vi "Set VI Ref.vi"(0 "reference in":refnum<class "Generic Utilities.lvclass">, 5 "error in (no error)":errorcluster, 6 "ReInit All to Default?":bool, 7 "GUI VI Ref":refnum<vi>, 8 "Initialize FP Control Refs":bool, 9 "Version #":string) -> (14 "reference out":refnum<class "Generic Utilities.lvclass">, 19 "error out":errorcluster)   [LabVIEW 2022 SP3, in "Generic Utilities.lvclass"]
uses:
  Generic Utilities.lvclass
  utils/FP Refnums.ctl
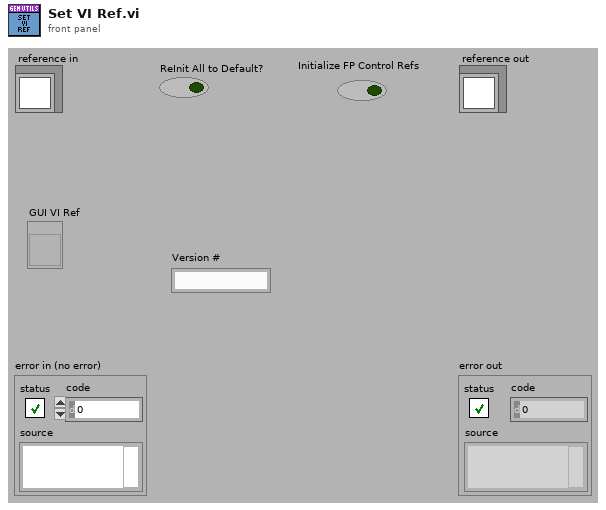
[diagram p1: front panel]
types:
  T1 = typedef "Generic Utilities.lvclass/FP Refnums.ctl" = cluster{"Panel refnum":refnum<vi>, "Control Labels":string[], "Refnums":refnum<vi>[]}
  T2 = typedef "Generic Utilities.lvclass/ObjectAttributesRef.ctl" = refnum<data-value>
  T3 = typedef "Generic Utilities.lvclass/ObjectAttributes.ctl" = cluster{"GUI Parameters":T4, "State Machine Control":cluster{"Timeout":i32, "State Queue":string[], "State History":string[], "State History Length":i32}, "Logging File Path":path, "OBJ not a refnum?":bool, "Timer Start":timestamp, "FP Refnums":T1}
  T4 = typedef "Generic Utilities.lvclass/GUI Parameters.ctl" = cluster{"Application Name":string, "GUI VI Ref":refnum<vi>, "Close Panel?":bool, "Message Window ref":refnum<vi>, "Version #":string}
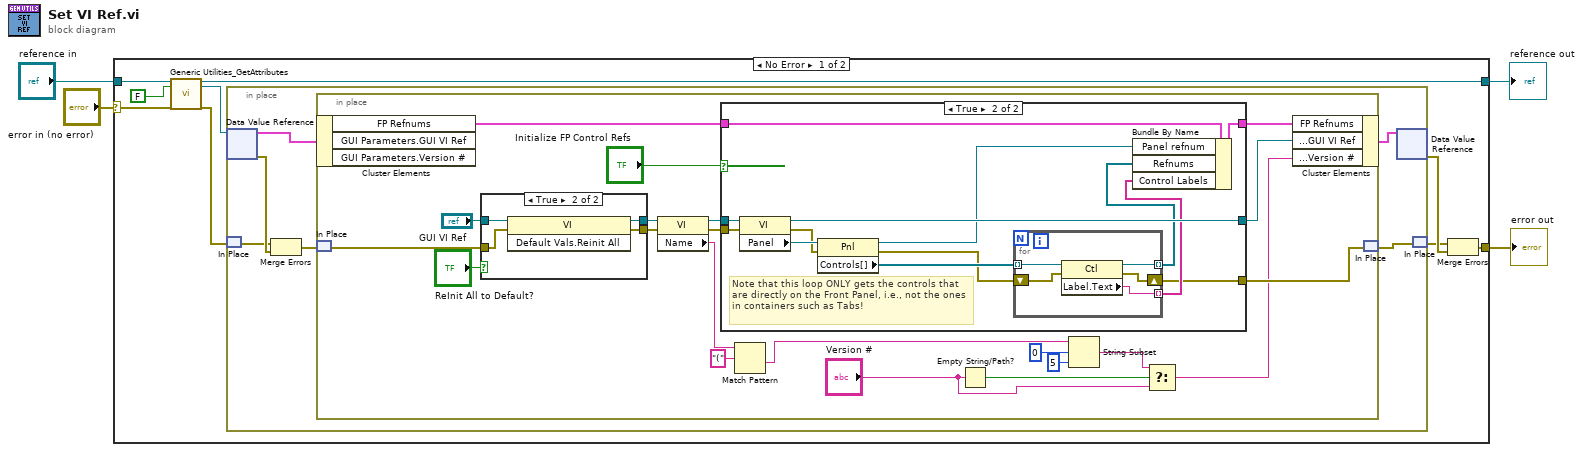
[diagram p0: block diagram]
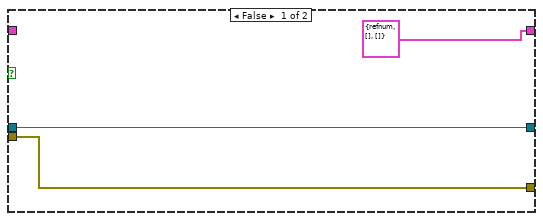
[diagram p2: hidden frame]
diagram:
  n1 = case shown="No Error" "error in (no error)" {
    selector: "error in (no error)" -> [w9 w69]
    tunnel: [w13 w69] -> w3
    tunnel: [w8 w68] -> w1
    tunnel: "reference in" -> [w11 w68]
    frame No Error {
      n2 = call "Generic Utilities_GetAttributes.vi"("reference in"=w11, "return data? (T)"=FALSE, "error in (no error)"=w9) -> ("reference out"=w8:refnum<class "Generic Utilities.lvclass">, "attributes ref"=w7:T2, "error out"=w6:errorcluster)  [unwired: 13 in, 1 out]
      n3 = in-place {
        n4 = in-place-dvr #1(w7) -> (w18:T3, w17:errorcluster)
        n5 = in-place-match #2(w6) -> (w16:errorcluster)
        n6 = Merge Errors(w16, w17) -> (w15:errorcluster)
        n7 = in-place {
          n8 = in-place-cluster #3(w18) -> ("FP Refnums"=w33:T1)  [unwired: 2 out]
          n9 = in-place-match #4(w15) -> (w38:errorcluster)
          n10 = case shown="True" "ReInit All to Default?" {
            tunnel: "GUI VI Ref" -> [w63 w67]
            tunnel: [w63 w66] -> w29
            tunnel: w38 -> [w62 w65]
            tunnel: [w62 w64] -> w27
            frame False {
            }
            frame True {
              n11 = invoke class="VI" method="Default Vals.Reinit All"(reference=w67, error in=w65) -> (reference out=w66:refnum<vi>, error out=w64:errorcluster)  [unwired: 1 in, 1 out]
            }
          }
          n12 = property class="VI"(reference=w29, error in=w27) -> (reference out=w28:refnum<vi>, error out=w26:errorcluster, "Name"=w25:string)
          n13 = case shown="True" "Initialize FP Control Refs" {
            tunnel: w28 -> [w43 w56]
            tunnel: w26 -> [w42 w55]
            tunnel: [w42 w45] -> w37
            tunnel: [w43 w50] -> w35
            tunnel: [T1 {"Panel refnum"=refnum, "Control Labels"=[], "Refnums"=[]} ("FP Refnums") w48] -> w34
            tunnel: w33 -> [_ w49]
            frame False {
            }
            frame True {
              # "Note that this loop ONLY gets the controls that are directly on the Front Panel, i.e., not the ones in containers such as Tabs!"
              n14 = property class="VI"(reference=w56, error in=w55) -> (reference out=w50:refnum<vi>, error out=w53:errorcluster, "Panel"=w54:refnum<vi>)
              n15 = property class="Pnl"(reference=w54, error in=w53) -> (reference out=w44:refnum<vi>, error out=w51:errorcluster, "Controls[]"=w52:refnum<vi>[])
              n16 = for {
                tunnel: w52 -> [w59] mode=indexing
                shift-right: [w60] -> w45
                shift-left: w51 -> [w61]
                tunnel: [w58] -> w47 mode=indexing
                tunnel: [w57] -> w46 mode=indexing
                n17 = property class="Ctl"(reference=w59, error in=w61) -> (reference out=w58:refnum<vi>, error out=w60:errorcluster, "Label.Text"=w57:string)
              }
              n18 = Bundle By Name(cluster=w49, "Panel refnum"=w44, "Refnums"=w47, "Control Labels"=w46) -> (w48:T1)
            }
          }
          n19 = Match Pattern(string=w25, regular expression="(") -> (after substring=w20:string)  [unwired: 1 in, 3 out]
          n20 = Empty String/Path?(string/path="Version #") -> (empty?=w32:bool)
          n21 = String Subset(string=w20, offset (0)=0, length (rest)=5 ("length (rest)")) -> (substring=w21:string)
          n22 = Select(t=w21, s=w32, f="Version #") -> (s? t:f=w30:string)
          n23 = in-place-cluster #3("FP Refnums"=w34, "GUI Parameters.GUI VI Ref"=w35, "GUI Parameters.Version #"=w30) -> (w19:T3)
          n24 = in-place-match #4(w37) -> (w14:errorcluster)
        }
        n25 = in-place-dvr #1(w19) -> (w12:errorcluster)  [unwired: 1 out]
        n26 = in-place-match #2(w14) -> (w5:errorcluster)
      }
      n27 = Merge Errors(w5, w12) -> (w13:errorcluster)
    }
    frame Error {
    }
  }
  "error out" <- w3
  "reference out" <- w1
